vi "prgpsu.vi"() -> ()   [LabVIEW 2012]
uses:
  <vilib>/Instr/_visa.llb/VISA Configure Serial Port (Instr).vi
panel:
  out "电流ascii":string
  out "电压ascii":string
  out "电流回显":dbl
  in  "模拟条":bool
  in  "电压":dbl min=0.0 max=60.0
  in  "电流":dbl min=0.0 max=5.0
  out "电压回显":dbl
  in  "电压":dbl(slide) scale=0.0..60.0 scale format="%.1g"
  in  "电流":dbl(slide) scale=0.0..5.0 scale format="%.1g"
  in  "停止":bool
  in  "VISA resource name":refnum<visa-resource-name> caption="VISA资源名称"
  in  "baud rate (9600)":u32=9600 caption="波特率(9600)"
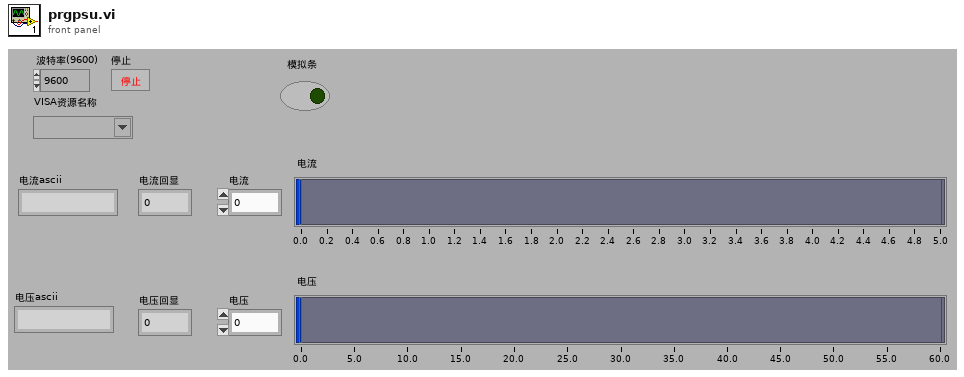
[diagram p1: front panel]
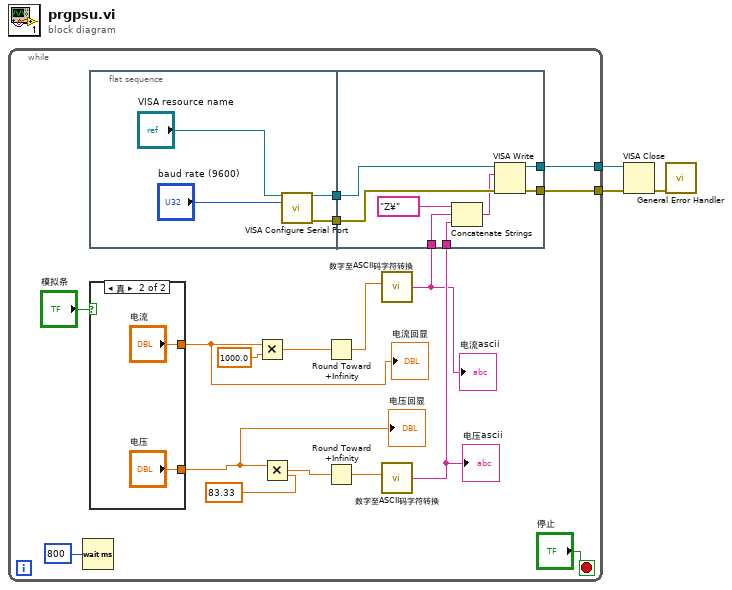
[diagram p0: block diagram]
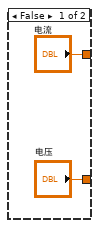
[diagram p2: hidden frame]
diagram:
  n1 = while {
    tunnel: [w11] -> w2
    tunnel: [w12] -> w1
    stop <- "停止" stop-if-true
    n2 = Wait (ms)(milliseconds to wait=u32 800 ("等待时间（毫秒）")) -> ()  [unwired: 1 out]
    n3 = flat-sequence {
      tunnel: [w27] -> w20
      tunnel: [w26] -> w19
      tunnel: w20 -> [w36]
      tunnel: w19 -> [w35]
      tunnel: w4 -> [w33]
      tunnel: w13 -> [w32]
      tunnel: [w30] -> w12
      tunnel: [w29] -> w11
      frame #0 {
        n4 = call-poly "VISA Configure Serial Port"("VISA resource name"="VISA resource name", "baud rate (9600)"="baud rate (9600)") -> ("VISA resource name out"=w26:refnum<visa-resource-name>, "error out"=w27:errorcluster)  [unwired: 4 in, 8 out]
      }
      frame #1 {
        n5 = Concatenate Strings("Z¥" ("写入缓冲区"), w33, w32) -> (w31:string)
        n6 = VISA Write(VISA resource name=w35, write buffer=w31, error in (no error)=w36) -> (VISA resource name out=w30:refnum<visa-resource-name>, error out=w29:errorcluster)  [unwired: 1 out]
      }
    }
    n7 = case shown="真" "模拟条" {
      tunnel: ["电流" "电流"] -> w5
      tunnel: ["电压" "电压"] -> w7
      frame False {
      }
      frame True {
      }
    }
    "电压回显" <- w7
    "电流回显" <- w5
    n8 = Multiply(x=w5, y=1000.0) -> (x*y=w10:dbl)
    n9 = Multiply(x=w7, y=83.33) -> (x*y=w9:dbl)
    n10 = Round Toward +Infinity(x=w10) -> (ceil(x): smallest int >= x=w6:dbl)
    n11 = Round Toward +Infinity(x=w9) -> (ceil(x): smallest int >= x=w8:dbl)
    n12 = call "数字至ASCII码字符转换.vi"("数字"=w6) -> ("ASCII码字符串"=w4:string)  [unwired: 3 in]
    "电流ascii" <- w4
    n13 = call "数字至ASCII码字符转换.vi"("数字"=w8) -> ("ASCII码字符串"=w13:string)  [unwired: 3 in]
    "电压ascii" <- w13
  }
  n14 = VISA Close(VISA resource name=w1, error in (no error)=w2) -> (error out=w3:errorcluster)
  n15 = call <vilib>:"General Error Handler.vi"("error in (no error)"=w3) -> ()  [unwired: 1 in, 14 out]
